vi "set_intensity_modifier.vi"(8 "error in (no error)":errorcluster, 10 "write signals":refnum<class "GenericSignalWriter.lvclass">, 11 "DL090202ScanHead.lvclass in":refnum<class "ScanHeadDL090202.lvclass">) -> (0 "error out":errorcluster, 3 "DL090202ScanHead.lvclass out":refnum<class "ScanHeadDL090202.lvclass">)   [LabVIEW 2010, in "ScanHeadDL090202.lvclass"]
uses:
  ScanHeadDL090202.lvclass
  SignalWriter/GenericSignalWriter/GenericSignalWriter/GenericSignalWriter.lvclass
  ScanHeadDL090202.lvclass/ScanHeadDL090202.ctl
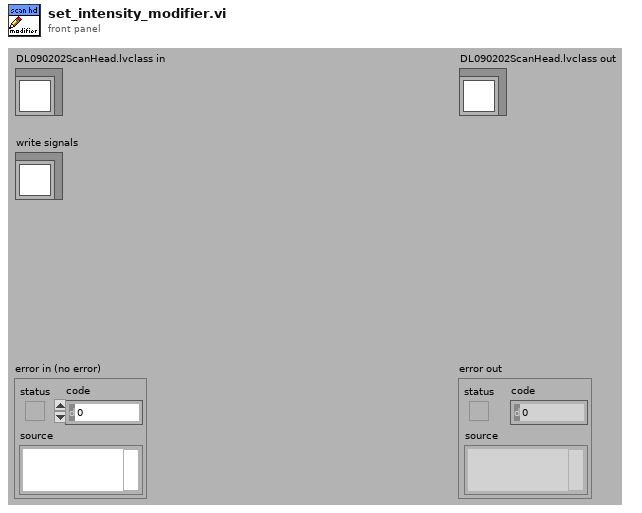
[diagram p1: front panel]
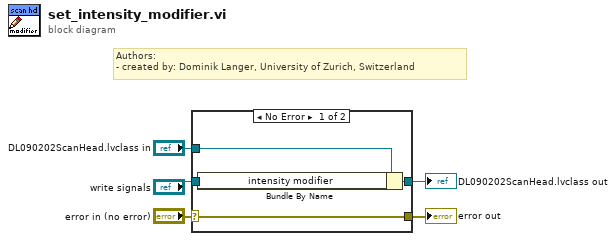
[diagram p0: block diagram]
diagram:
  # "Authors: \n- created by: Dominik Langer, University of Zurich, Switzerland"
  n1 = case shown="No Error" "error in (no error)" {
    selector: "error in (no error)" -> [w9 w10]
    tunnel: [w9 w10] -> w4
    tunnel: [w7 w11] -> w2
    tunnel: "DL090202ScanHead.lvclass in" -> [w8 w11]
    tunnel: "write signals" -> [w6 _]
    frame No Error {
      n2 = Bundle By Name(cluster=w8, "intensity modifier"=w6) -> (w7:refnum<class "ScanHeadDL090202.lvclass">)
    }
    frame Error {
    }
  }
  "error out" <- w4
  "DL090202ScanHead.lvclass out" <- w2
